vi "www template engine.vi"(10 "Template Dictionary (empty)":T1, 11 "Template String (\"\")":string) -> (2 "dup Template Dictionary":T1, 3 "Template String out":string)   [LabVIEW 2011]
uses:
  ITK EXT/utils/keyedarr.llb/Keyed Array.ctl
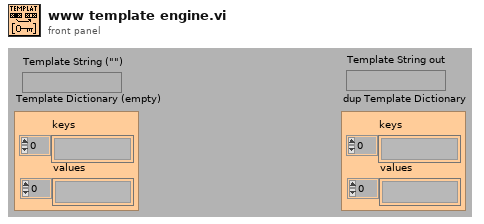
[diagram p1: front panel]
types:
  T1 = typedef "Keyed Array.ctl" = cluster{"keys":string[], "values":string[]}
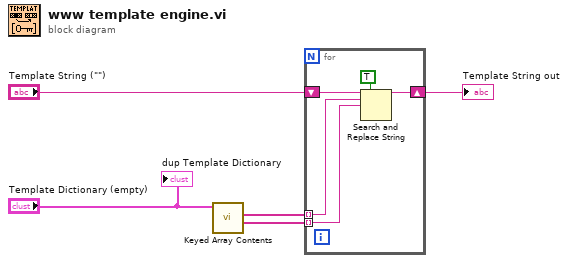
[diagram p0: block diagram]
diagram:
  n1 = call "Keyed Array Contents.vi"("array in"="Template Dictionary (empty)") -> ("values"=w4:string[], "keys"=w5:string[])  [unwired: 5 out]
  n2 = for {
    shift-right: [w8] -> w2
    shift-left: "Template String (\"\")" -> [w9]
    tunnel: w5 -> [w7] mode=indexing
    tunnel: w4 -> [w6] mode=indexing
    n3 = Search and Replace String(replace all?=TRUE, input string=w9, search string=w7, replace string=w6) -> (result string=w8:string)  [unwired: 1 in, 6 out]
  }
  "Template String out" <- w2
  "dup Template Dictionary" <- "Template Dictionary (empty)"
